vi "etc_XCITE_GetDeviceInfo.vi"(0 "h":u64, 5 "error in (no error)":errorcluster {"code" format="%x"}) -> (14 "h out":u64, 15 "ErrorMessage":i32 format="%x", 16 "type":i32(ring)=65535 items=["XC_120PC"=0, "XC_exacte"=1, "XC_120LED"=2, "XC_110LED"=3, "XC_mini"=4, "XC_XYLIS"=5, "XC_XR210"=6, "XC_LED1"=7, "XC_XT600"=8, "XC_XT900"=9, "Any"=65535], 17 "port":string, 18 "open_count":u32, 19 "error out":errorcluster {"code" format="%x"})   [LabVIEW 2019, in "XCite.lvlib"]
doc: "Get information about the slelected X-cite device."
uses:
  XCite.lvlib
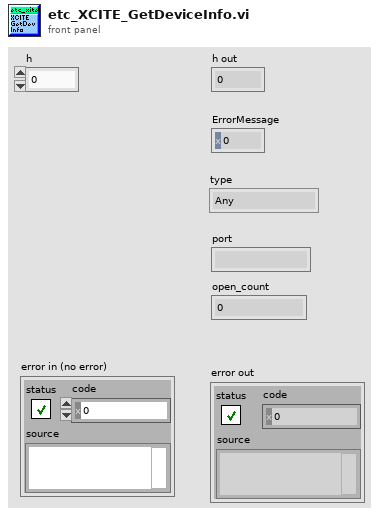
[diagram p1: front panel]
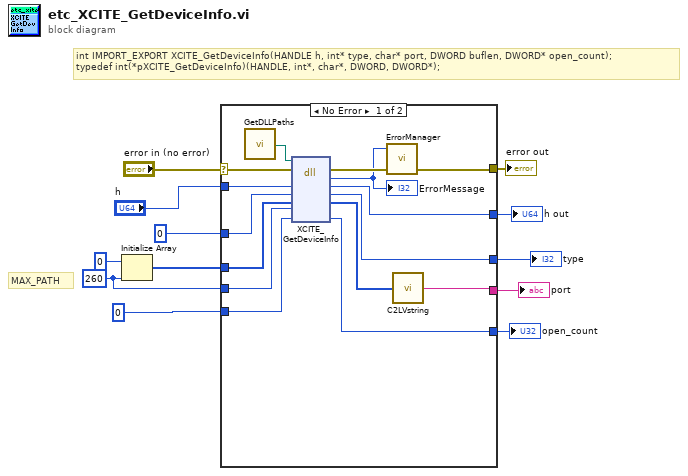
[diagram p0: block diagram]
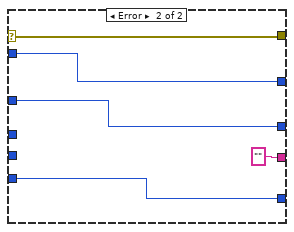
[diagram p2: hidden frame]
diagram:
  w3 = u16 260 ("dimension size")
  # "MAX_PATH"
  # "int IMPORT_EXPORT XCITE_GetDeviceInfo(HANDLE h, int* type, char* port, DWORD buflen, DWORD* open_count);\ntypedef int(*pXCITE_GetDeviceInfo)(HANDLE, int*, char*, DWORD, DWORD*);"
  n1 = Initialize Array(u8 0, w3) -> (w2:u8[])
  n2 = case shown="No Error" "error in (no error)" {
    selector: "error in (no error)" -> [w27 w32]
    tunnel: [w25 w32] -> w12
    tunnel: "h" -> [w23 w31]
    tunnel: [w22 w31] -> w10
    tunnel: w3 -> [w20 _]
    tunnel: [w13 "" ("string")] -> w5
    tunnel: u32 0 ("open_count") -> [w19 w30]
    tunnel: [w18 w30] -> w7
    tunnel: 0 ("type") -> [w17 w29]
    tunnel: [w16 w29] -> w1
    tunnel: w2 -> [w15 _]
    frame No Error {
      n3 = call "GetDLLPaths.vi"() -> ("etc_xcite_path"=w21:path)  [unwired: 8 in, 3 out]
      n4 = dll-call lib="C:/LabVIEWDevFall2024/pco.labview/labview_sdk/runtime/bin64/etc_xcite.dll" fn="XCITE_GetDeviceInfo"(path in=w21, error in=w27, "h"=w23, "type"=w17, "port"=w15, "buflen"=w20, "open_count"=w19) -> (error out=w26:errorcluster, "return type"=w24:i32, "h"=w22:u64, "type"=w16:i32, "port"=w14:u8[], "open_count"=w18:u32)  [unwired: 2 in, 1 out]
      "ErrorMessage" <- w24
      n5 = call "ErrorManager.vi"("error in (no error)"=w26, "error code"=w24) -> ("error out"=w25:errorcluster)  [unwired: 2 in, 1 out]
      n6 = call "C2LVstring.vi"("CString"=w14) -> ("LVString"=w13:string)  [unwired: 4 in]
    }
    frame Error {
    }
  }
  "error out" <- w12
  "h out" <- w10
  "open_count" <- w7
  "port" <- w5
  "type" <- w1
